vi "mbdmaboot_Host.vi"() -> ()   [LabVIEW 2015]
uses:
  <vilib>/FPGAPlugInAG/USRP X310; 294xR; 295xR/niLvFpga_Open_USRP X310; 294xR; 295xR.vi
  <vilib>/rvi/interface/common/dynamic/niFpgaDynamicAddResources.vi
  <vilib>/FPGAPlugInAG/Dynamic/niLvFpga_Download_Dynamic.vi
  <vilib>/FPGAPlugInAG/Dynamic/niLvFpga_Run_Dynamic.vi
  <vilib>/Utility/error.llb/Error Cluster From Error Code.vi
  <vilib>/rvi/errors/niLvFpgaAdjustHostInterfaceError.vi
  <vilib>/FPGAPlugInAG/Dynamic/niLvFpga_Close_Dynamic.vi
  <vilib>/rvi/interface/nirviOpenFPGA/nirviOpenFPGA.xnode
  FPGA Bitfiles/mb-dmaboot_FPGATarget_mbdmaboottopLeve_XKhxGc+VYWY.lvbitx
  <vilib>/rvi/interface/nirviMethod/nirviMethod.xnode
  <vilib>/rvi/interface/nirviReadWriteControl/nirviReadWriteControl.xnode
  <vilib>/rvi/interface/nirviCloseFPGA/nirviCloseFPGA.xnode
  <vilib>/FPGAPlugInAG/Dynamic/niLvFpga_ReadFifo_Dynamic.vi
  <vilib>/rvi/errors/niLvFpgaMergeErrorWithErrorCode.vi
  NiFpgaLv.dll
  <vilib>/rvi/interface/Simulation/niFpgaSimulationCallBeginRW.vi
  <vilib>/FPGAPlugInAG/Dynamic/niLvFpga_WriteFifo_Dynamic.vi
panel:
  out "Console out (readonly) 2":string="FPGA is done configure. No software running.\nÿ"
  out "C":u32
  in  "B":u32
  in  "A":u32
  out "Done":bool
  in  "Elf File to Download:":path=path "xsdk_worspace/helloworld1/Debug/helloworld1.elf"
  in  "Download ELF file":bool
  in  "stop":bool
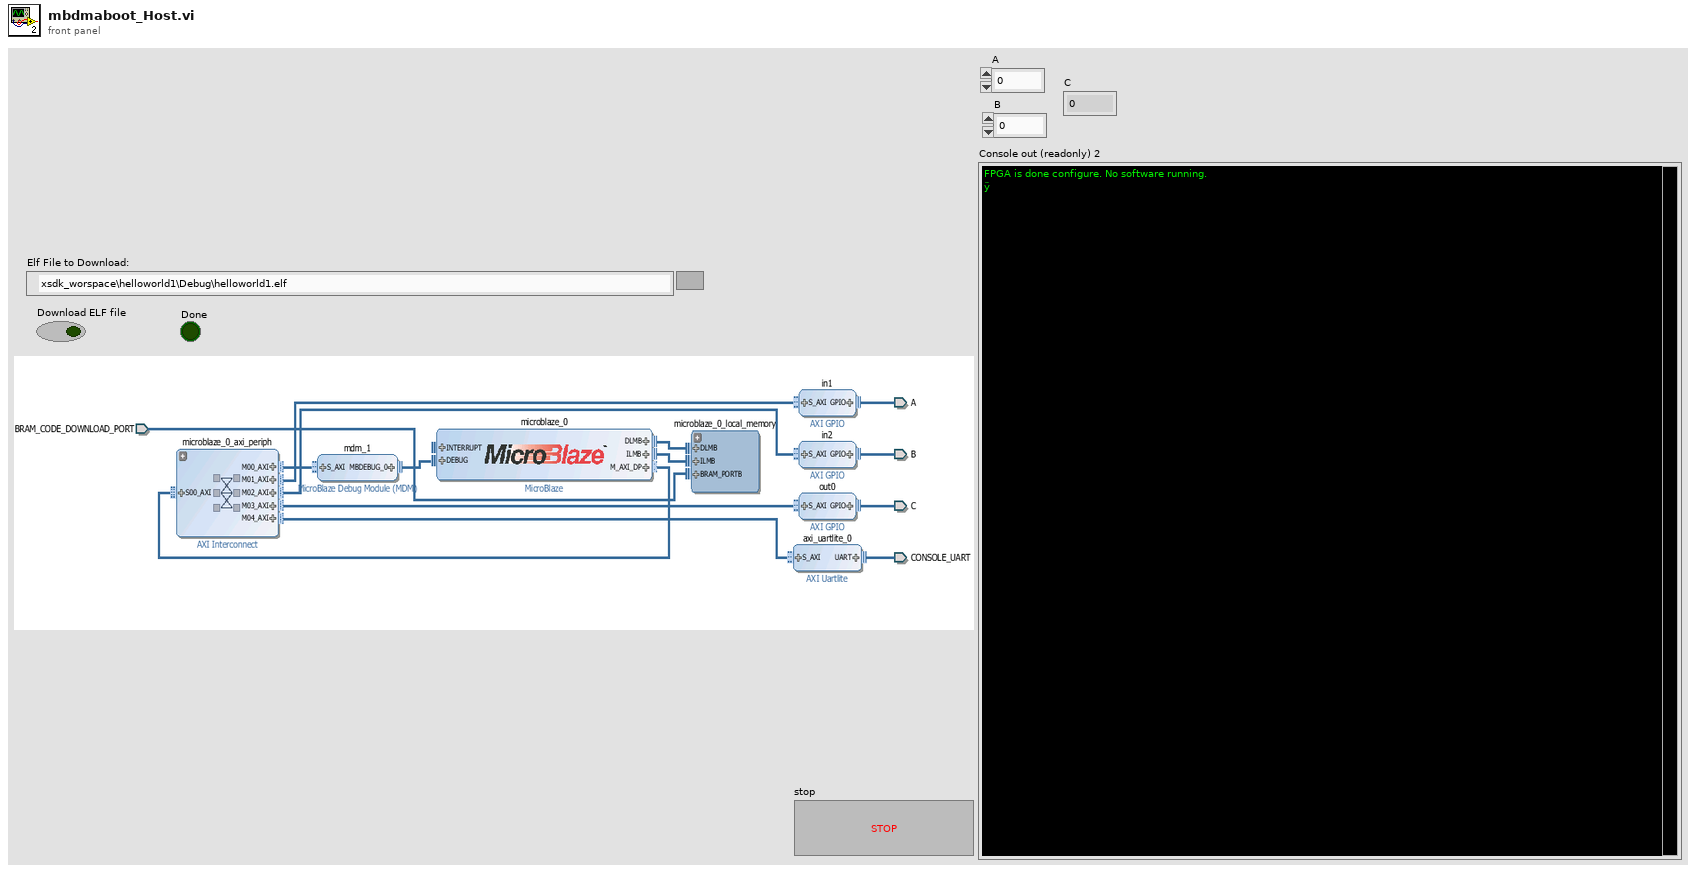
[diagram p1: front panel]
types:
  T1 = typedef "DataControl.ctl" = cluster{"Address":u32, "Data":u32}[]
  T2 = cluster{"Baud (ticks)":u32, "CharacterSize":u8, "Parity":enum8{"None", "Even", "Odd"}, "Stop Bits":enum8{"1.0", "1.5", "2.0"}, "Spacing (ticks)":u32}
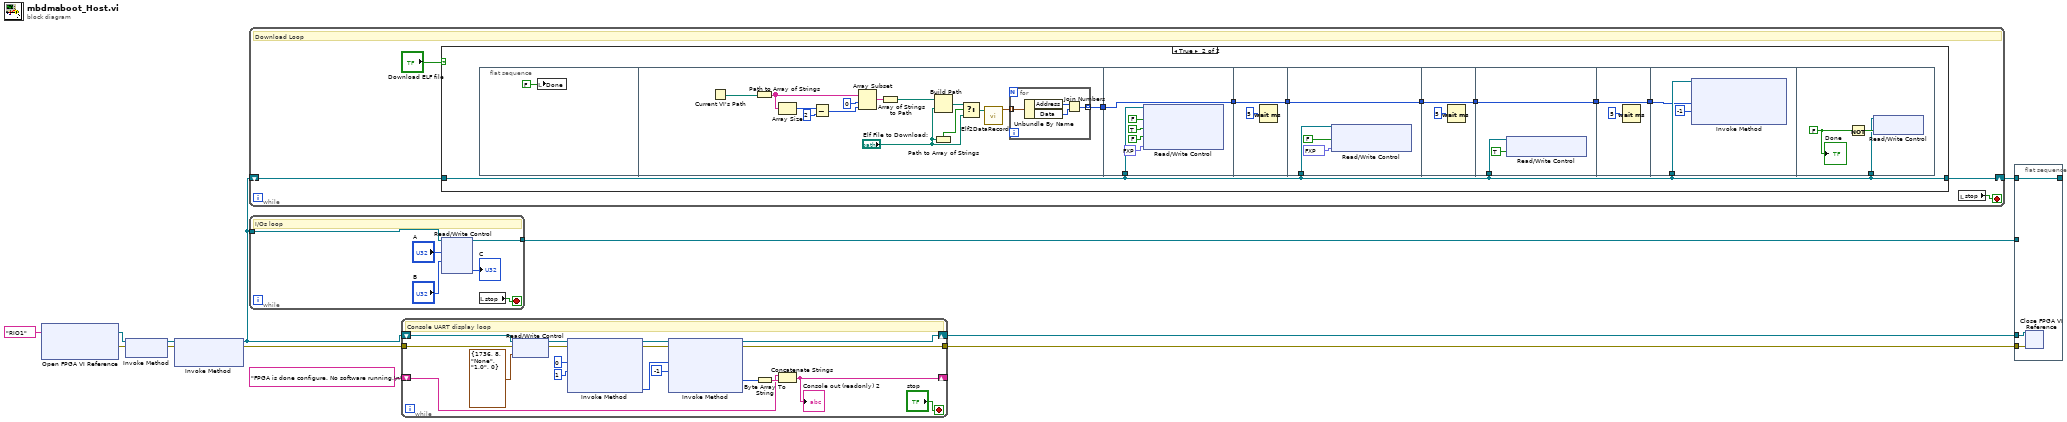
[diagram p0: block diagram]
diagram:
  n1 = xnode "Open FPGA VI Reference"("resource name"=tag "RIO1") -> ("FPGA VI Reference Out"=w12:refnum<k20>, "error out"=w10:errorcluster)  [unwired: 1 in]
  n2 = xnode "Invoke Method"("FPGA VI Reference In"=w12, "error in"=w10) -> ("FPGA VI Reference Out"=w11:refnum<k20>, "error out"=w9:errorcluster)
  n3 = xnode "Invoke Method"("FPGA VI Reference In"=w11, "error in"=w9) -> ("FPGA VI Reference Out"=w2:refnum<k20>, "error out"=w7:errorcluster)  [unwired: 1 in]
  n4 = while {
    shift-right: [w13] -> w3
    shift-left: w2 -> [w14]
    stop <- w16 stop-if-true
    # "Download Loop"
    n5 = case shown="True" "Download ELF file" {
      tunnel: w14 -> [w17 w18]
      tunnel: [w17 w18] -> w13
      frame False {
      }
      frame True {
        n6 = flat-sequence {
          tunnel: [w39] -> w25
          tunnel: w25 -> [w50]
          tunnel: [w50] -> w24
          tunnel: w18 -> [w49]
          tunnel: w24 -> [w52]
          tunnel: [w52] -> w23
          tunnel: w23 -> [w56]
          tunnel: [w56] -> w22
          tunnel: w18 -> [w55]
          tunnel: w22 -> [w58]
          tunnel: [w58] -> w21
          tunnel: w21 -> [w61]
          tunnel: [w61] -> w20
          tunnel: w18 -> [w59]
          tunnel: w20 -> [w63]
          tunnel: [w63] -> w19
          tunnel: w19 -> [w65]
          tunnel: w18 -> [w66]
          tunnel: w18 -> [w67]
          frame #0 {
            n7 = local write "Done"(FALSE ("Done")) -> ()
          }
          frame #1 {
            n8 = Current VI's Path() -> (path=w32:path)
            n9 = Path to Array of Strings(0:w32) -> (2:w37:string[])  [unwired: 1 out]
            n10 = Array Size(array=w37) -> (size(s)=w35:i32)
            n11 = Subtract(x=w35, y=2) -> (x-y=w36:i32)
            n12 = Array Subset(array=w37, index=0, length=w36) -> (w33:string[])
            n13 = Array of Strings to Path(0:w33) -> (2:w31:path)  [unwired: 1 in]
            n14 = Path to Array of Strings(0:"Elf File to Download:") -> (1:w30:bool)  [unwired: 1 out]
            n15 = Build Path(base path=w31, name or relative path="Elf File to Download:") -> (appended path=w28:path)
            n16 = Select(t=w28, s=w30, f="Elf File to Download:") -> (s? t:f=w27:path)
            n17 = call "Elf2DataRecord.vi"("Elf file"=w27) -> ("DataRecord"=w40:T1)  [unwired: 10 in]
            n18 = for {
              tunnel: w40 -> [w44] mode=indexing
              tunnel: [w41] -> w39 mode=indexing
              n19 = Unbundle By Name(w44) -> ("Address"=w43:u32, "Data"=w42:u32)
              n20 = Join Numbers(hi=w43, lo=w42) -> ((hi.lo)=w41:u64)
            }
          }
          frame #2 {
            n21 = xnode "Read/Write Control"("FPGA VI Reference In"=w49, "ub1\\reset_rtl"=FALSE ("ub1\\reset_rtl"), "ub1\\BRAM_PORTB_rst"=TRUE ("ub1\\BRAM_PORTB_rst"), "ub1\\BRAM_PORTB_en"=FALSE ("ub1\\BRAM_PORTB_en"), "ub1\\BRAM_PORTB_we"=fxp<+,4,4> 0.0 ("ub1\\BRAM_PORTB_we")) -> ()  [unwired: 1 in, 2 out]
          }
          frame #3 {
            n22 = Wait (ms)(milliseconds to wait=u32 5) -> ()  [unwired: 1 out]
          }
          frame #4 {
            n23 = xnode "Read/Write Control"("FPGA VI Reference In"=w55, "ub1\\BRAM_PORTB_rst"=FALSE ("ub1\\BRAM_PORTB_en"), "ub1\\BRAM_PORTB_we"=fxp<+,4,4> 15.0 ("ub1\\BRAM_PORTB_we")) -> ()  [unwired: 1 in, 2 out]
          }
          frame #5 {
            n24 = Wait (ms)(milliseconds to wait=u32 5) -> ()  [unwired: 1 out]
          }
          frame #6 {
            n25 = xnode "Read/Write Control"("FPGA VI Reference In"=w59, "ub1\\BRAM_PORTB_en"=TRUE ("ub1\\BRAM_PORTB_en")) -> ()  [unwired: 1 in, 2 out]
          }
          frame #7 {
            n26 = Wait (ms)(milliseconds to wait=u32 5) -> ()  [unwired: 1 out]
          }
          frame #8 {
            n27 = xnode "Invoke Method"("FPGA VI Reference In"=w66, "Data"=w65, "Timeout (ms)"=-1) -> ()  [unwired: 1 in, 3 out]
          }
          frame #9 {
            w69 = FALSE
            n28 = Not(x=w69) -> (.not. x?=w68:bool)
            n29 = xnode "Read/Write Control"("FPGA VI Reference In"=w67, "ub1\\reset_rtl"=w68) -> ()  [unwired: 1 in, 2 out]
            "Done" <- w69
          }
        }
      }
    }
    n30 = local read "stop"() -> (w16:bool)
  }
  n31 = while {
    tunnel: w2 -> [w75]
    tunnel: [w70] -> w1
    stop <- w71 stop-if-true
    # "I/Os loop"
    n32 = xnode "Read/Write Control"("FPGA VI Reference In"=w75, "A"="A", "B"="B") -> ("FPGA VI Reference Out"=w70:refnum<k20>, "C"=→"C":u32)  [unwired: 1 in, 1 out]
    n33 = local read "stop"() -> (w71:bool)
  }
  n34 = while {
    shift-right: [w86] -> w8
    shift-left: w2 -> [w93]
    tunnel: w7 -> [w82]
    tunnel: [w87] -> w6
    shift-right: [w78] -> _
    shift-left: "FPGA is done configure. No software running.\n" ("string") -> [w76]
    stop <- "stop" stop-if-true
    # "Console UART display loop"
    n35 = xnode "Read/Write Control"("FPGA VI Reference In"=w93, "error in"=w82, "Settings"=T2 {"Baud (ticks)"=1736, "CharacterSize"=8, "Parity"=enum."None", "Stop Bits"=enum."1.0", "Spacing (ticks)"=0}) -> ("FPGA VI Reference Out"=w83:refnum<k20>, "error out"=w81:errorcluster)
    n36 = xnode "Invoke Method"("FPGA VI Reference In"=w83, "error in"=w81, "Number of Elements"=u32 0, "Timeout (ms)"=1) -> ("FPGA VI Reference Out"=w89:refnum<k20>, "error out"=w88:errorcluster, "Elements Remaining"=w85:u32)  [unwired: 1 out]
    n37 = xnode "Invoke Method"("FPGA VI Reference In"=w89, "error in"=w88, "Number of Elements"=w85, "Timeout (ms)"=-1) -> ("FPGA VI Reference Out"=w86:refnum<k20>, "error out"=w87:errorcluster, "Data"=w79:u16[])  [unwired: 1 out]
    n38 = Byte Array To String(unsigned byte array=w79) -> (string=w77:string)
    n39 = Concatenate Strings(w76, w77) -> (w78:string)
    "Console out (readonly) 2" <- w78
  }
  n40 = flat-sequence {
    tunnel: w8 -> [w96]
    tunnel: w6 -> [w95]
    tunnel: [w94] -> _
    tunnel: w3 -> [w94]
    tunnel: w1 -> [_]
    frame #0 {
      n41 = xnode "Close FPGA VI Reference"("FPGA VI Reference In"=w96, "error in"=w95) -> ()  [unwired: 1 out]
    }
  }
